vi "ProdaNG.Tree.Process.Add.vi"(7 "Tree":refnum<vi>, 8 "error in (no error)":errorcluster, 9 "WabcoPartId":i32, 10 "ProcessStep":T1) -> (0 "error out":errorcluster)   [LabVIEW 2016]
uses:
  Controls/ProdaNG.Process.ctl
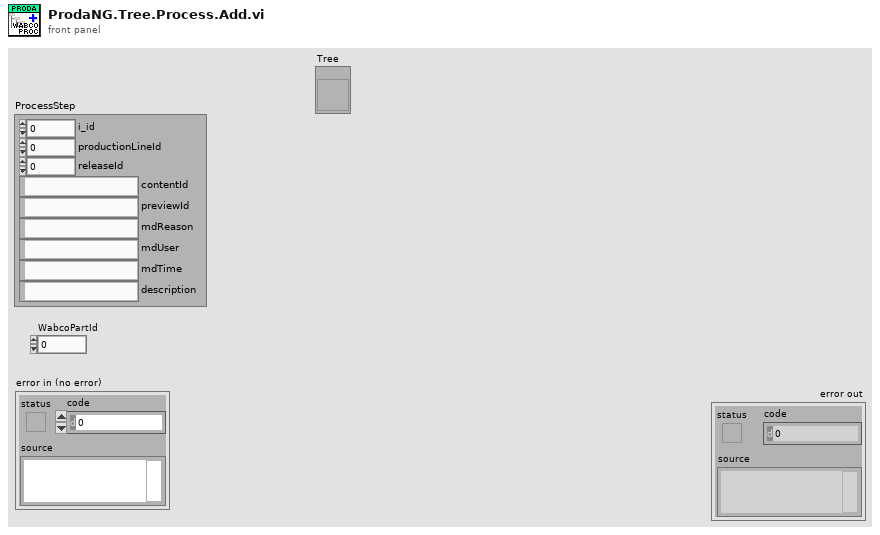
[diagram p1: front panel]
types:
  T1 = typedef "ProdaNG.Process.ctl" = cluster{"i_id":i32, "productionLineId":i32, "releaseId":i32, "contentId":string, "previewId":string, "mdReason":string, "mdUser":string, "mdTime":string, "description":string}
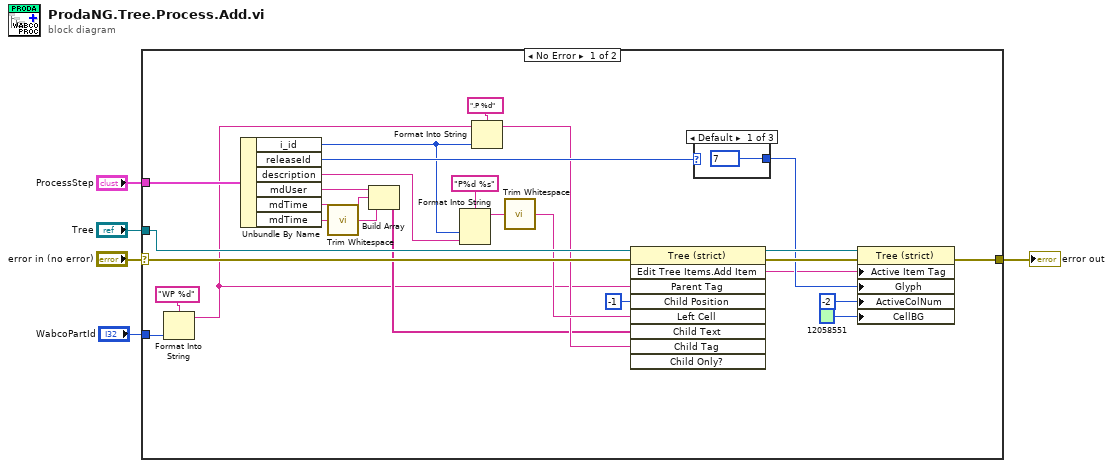
[diagram p0: block diagram]
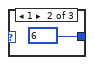
[diagram p2: hidden frame]
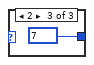
[diagram p3: hidden frame]
diagram:
  n1 = case shown="No Error" "error in (no error)" {
    selector: "error in (no error)" -> [w32 w36]
    tunnel: [w30 w36] -> w4
    tunnel: "Tree" -> [w31 _]
    tunnel: "ProcessStep" -> [w29 _]
    tunnel: "WabcoPartId" -> [w9 _]
    frame No Error {
      n2 = Format Into String(format string="WP %d", w9) -> (resulting string=w6:string)  [unwired: 2 in, 1 out]
      n3 = Unbundle By Name(w29) -> ("i_id"=w17:i32, "releaseId"=w27:i32, "description"=w28:string, "mdUser"=w12:string, "mdTime"=w7:string, "mdTime"=w11:string)
      n4 = call <vilib>:"Trim Whitespace.vi"("string"=w11) -> ("trimmed string"=w8:string)  [unwired: 1 in]
      n5 = Build Array(w12, w7, w8) -> (w10:string[])
      n6 = Format Into String(format string="P%d %s", w17, w28) -> (resulting string=w19:string)  [unwired: 2 in, 1 out]
      n7 = Format Into String(format string=".P %d", initial string=w6, w17) -> (resulting string=w15:string)  [unwired: 1 in, 1 out]
      n8 = call <vilib>:"Trim Whitespace.vi"("string"=w19) -> ("trimmed string"=w16:string)  [unwired: 1 in]
      n9 = invoke class="Tree (strict)" method="Edit Tree Items.Add Item"(reference=w31, error in=w32, "Parent Tag"=w6, "Child Position"=-1, "Left Cell"=w16, "Child Text"=w10, "Child Tag"=w15) -> (reference out=w24:refnum<vi>, error out=w25:errorcluster, "Edit Tree Items:Add Item"=w18:string)  [unwired: 2 in, 6 out]
      n10 = case shown="Default" w27 {
        tunnel: [7 6 7] -> w23
        frame Default {
        }
        frame 1 {
        }
        frame 2 {
        }
      }
      n11 = property class="Tree (strict)"(reference=w24, error in=w25, "Active Item Tag"=w18, "Glyph"=w23, "ActiveColNum"=-2 ("Active Cell:Active Column Number"), "CellBG"=u32 12058551) -> (error out=w30:errorcluster)  [unwired: 1 out]
    }
    frame Error {
    }
  }
  "error out" <- w4
